vi "load_xml.vi"(8 "error in":errorcluster, 10 "child node in":refnum<k20>) -> (0 "error out":errorcluster, 2 "child node out":refnum<k20>, 3 "HSDIO Settings":T1={"Enable HSDIO Pulses"=TRUE, "Resource Name"="PXI1Slot6", "Clock Rate"=20000000.0, "Array of Script Triggers"=[], "Pulse Generation Script"="script script1\n     Generate RedTrap_compress_temp\nend script", "Start Trigger"={"Wait for start trigger?"=FALSE, "source (PFI 0)"="PFI0", "edge (rising)"=12}, "Hardware alignment quantum\n(in samples)"=1, "Inital State"="", "Idle State"="", "Active Channels"="", "Array of Waveforms"=[]} {"Hardware alignment quantum\n(in samples)" min=1 step=1; "Array of Script Triggers"."level" items=["High Level"=34, "Low Level"=35]; "Array of Script Triggers"."edge" items=["Rising Edge"=12, "Falling Edge"=13]; "Start Trigger"."edge (rising)" items=["Rising Edge"=12, "Falling Edge"=13]; "Clock Rate" min=0.0 max=200000000.0 format="%.2p"})   [LabVIEW 2013, in "HSDIO.lvclass"]
doc: "Loads HSDIO settings from xml. Expected format:\n\n<EnableHSDIOPulses>%b</EnableHSDIOPulses>\n<ResourceName>%s</ResourceName>\n<ClockRate>%f</ClockRate>\n<unitsPerSecond>%f</unitsPerSecond>\n<HardwareAlignmentQuantum units=\"samples\">%u</HardwareAlignmentQuantum>\n<ArrayOfScriptTriggers columns=\"id, source, type, edge, level\">\n<trigger>%s\\t%s\\t%s\\t%s\\t%s</trigger>\n</ArrayOfScriptTriggers>\n<ChannelsControl columns=\"Description, Active?, Idle State\">\n<channel>%s</channel>\n</ChannelsControl>\n<PulseGenerationScript>%s</PulseGenerationScript>\n<DirectoryToLookForWaveformFiles>%s</DirectoryToLookForWaveformFiles>\n<StartTrigger.WaitForStartTrigger>%b</StartTrigger.WaitForStartTrigger>\n<StartTrigger.source>%s</StartTrigger.source>\n<StartTrigger.edge>%s</StartTrigger.edge>\n\nMTL 2013 Jan 1"
uses:
  HSDIO.lvclass
  <resource>/objmgr/DOMUserDefRef.rc
  <vilib>/xml/NI_XML.lvlib
  <vilib>/xml/Close Reference(Node).vi
  <instrlib>/niHSDIO/niHSDIO.llb/niHSDIO_ctl Trigger Script - trigID Values (Ring).ctl
  <instrlib>/niHSDIO/niHSDIO.llb/niHSDIO_ctl Trigger Source Values (Ring).ctl
  <instrlib>/niHSDIO/niHSDIO.llb/niHSDIO_ctl Trigger DigEdge - Edge Values (Ring).ctl
  <instrlib>/niHSDIO/niHSDIO.llb/niHSDIO_ctl Trigger DigLvl - Level Values (Ring).ctl
  HSDIO_settings.ctl
  waveform.ctl
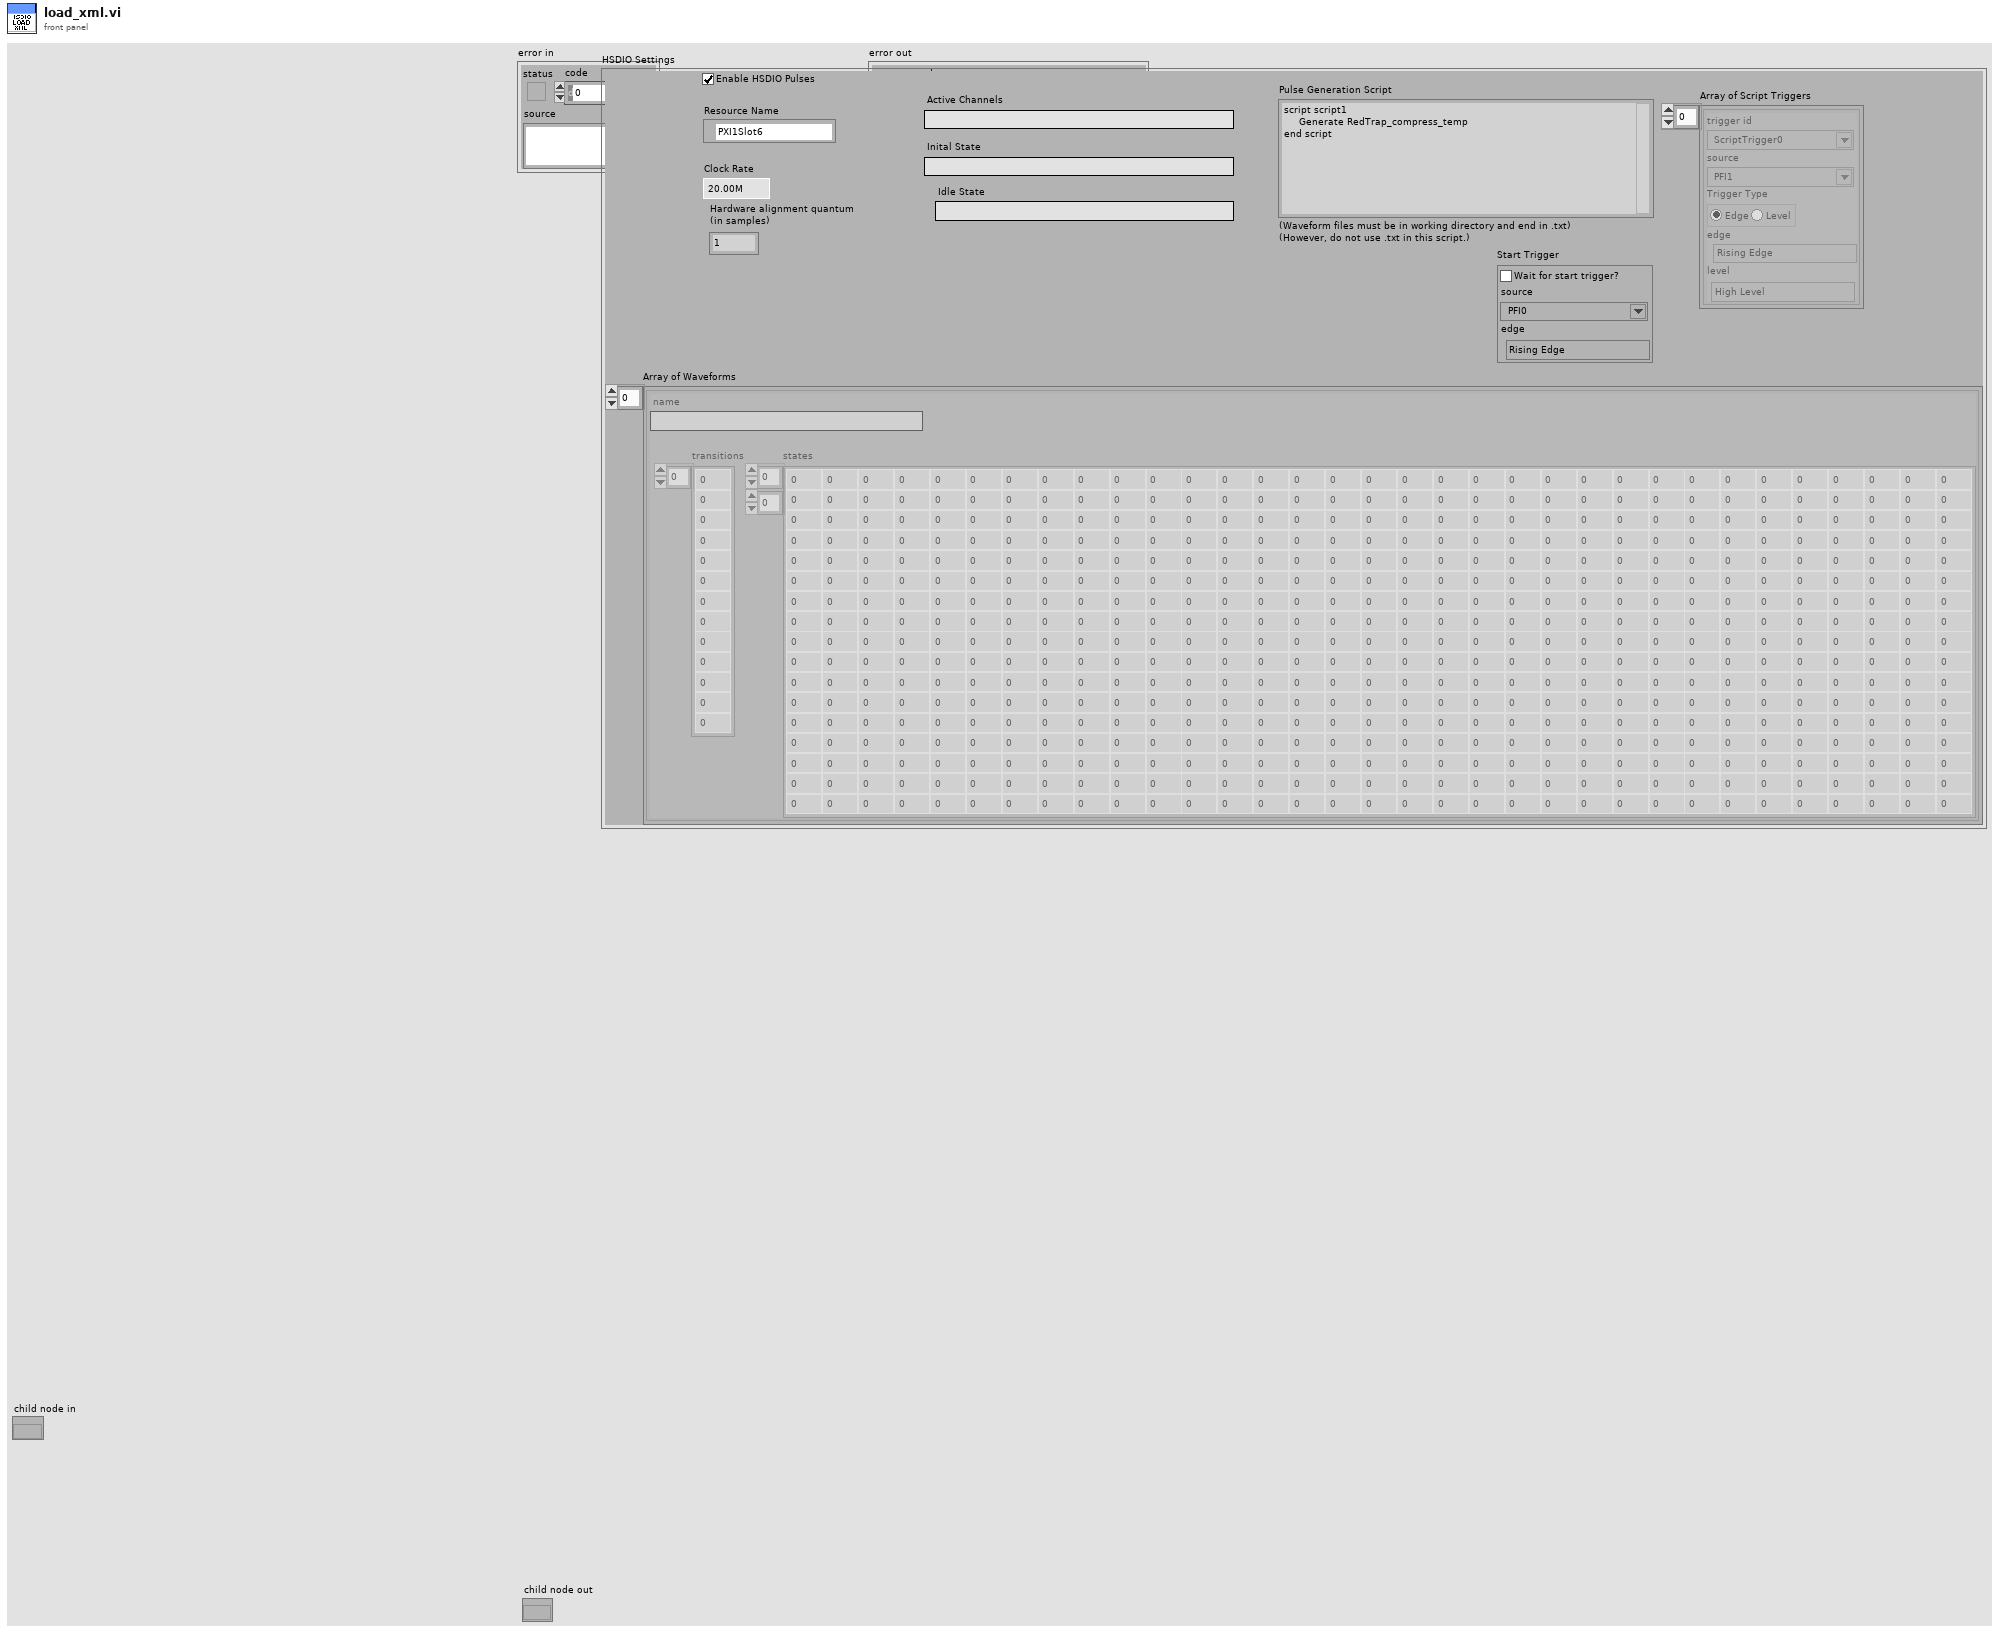
[diagram p1: front panel]
types:
  T1 = typedef "HSDIO.lvclass/HSDIO_settings.ctl" = cluster{"Enable HSDIO Pulses":bool, "Resource Name":refnum<k15>, "Clock Rate":dbl, "Array of Script Triggers":cluster{"trigger id (script trigger 0)":T2, "source (PFI 0)":T3, "Trigger Type":enum32{"Edge", "Level"}, "edge":T4, "level":T5}[], "Pulse Generation Script":string, "Start Trigger":cluster{"Wait for start trigger?":bool, "source (PFI 0)":T3, "edge (rising)":T4}, "Hardware alignment quantum\n(in samples)":u16, "Inital State":string, "Idle State":string, "Active Channels":string, "Array of Waveforms":T6[]}
  T2 = typedef "niHSDIO_ctl Trigger Script - trigID Values (Ring).ctl" = string
  T3 = typedef "niHSDIO_ctl Trigger Source Values (Ring).ctl" = string
  T4 = typedef "niHSDIO_ctl Trigger DigEdge - Edge Values (Ring).ctl" = i32
  T5 = typedef "niHSDIO_ctl Trigger DigLvl - Level Values (Ring).ctl" = i32
  T6 = typedef "HSDIO.lvclass/waveform.ctl" = cluster{"name":string, "transitions":u32[], "states":u8[][]}
  T7 = cluster{"trigger id (script trigger 0)":T2, "source (PFI 0)":T3, "Trigger Type":enum32{"Edge", "Level"}, "edge":T4, "level":T5}
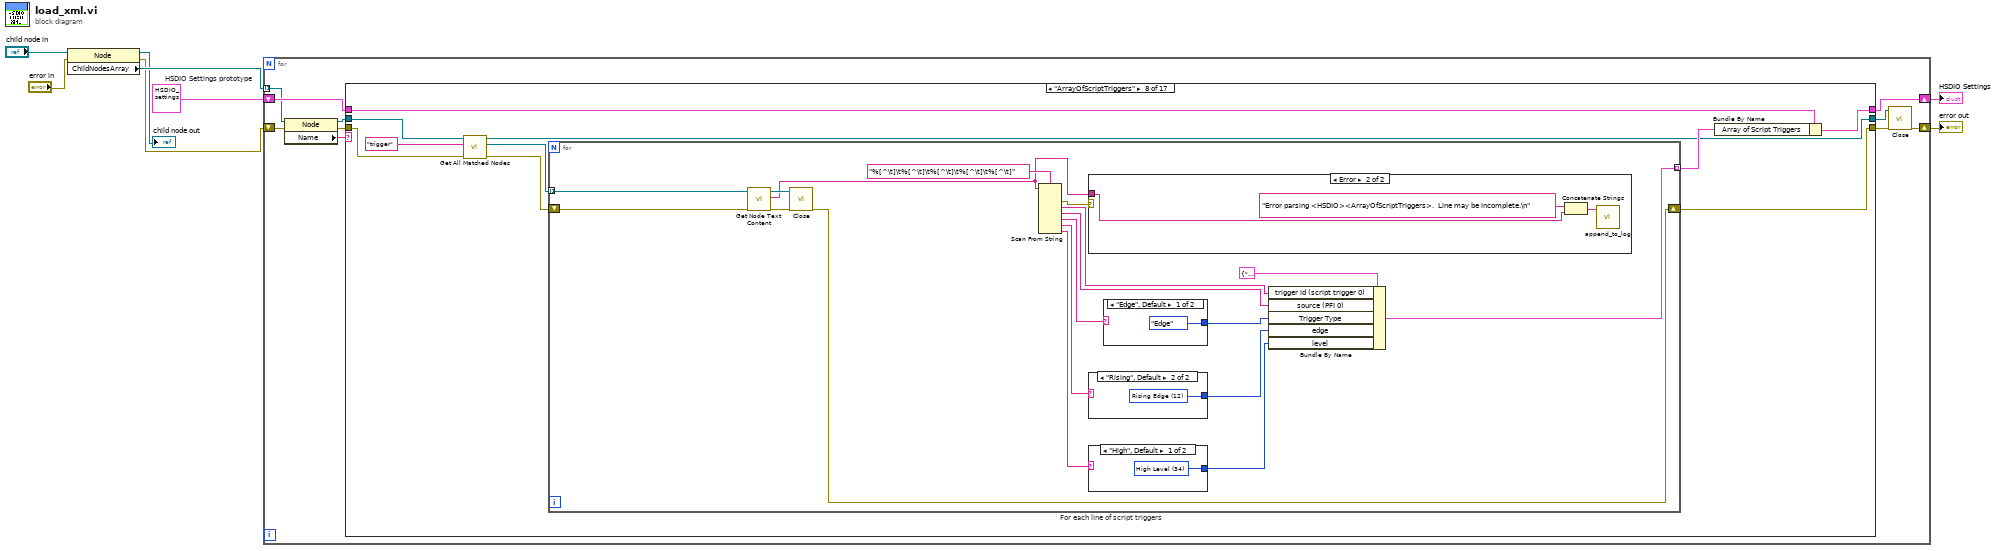
[diagram p0: block diagram]
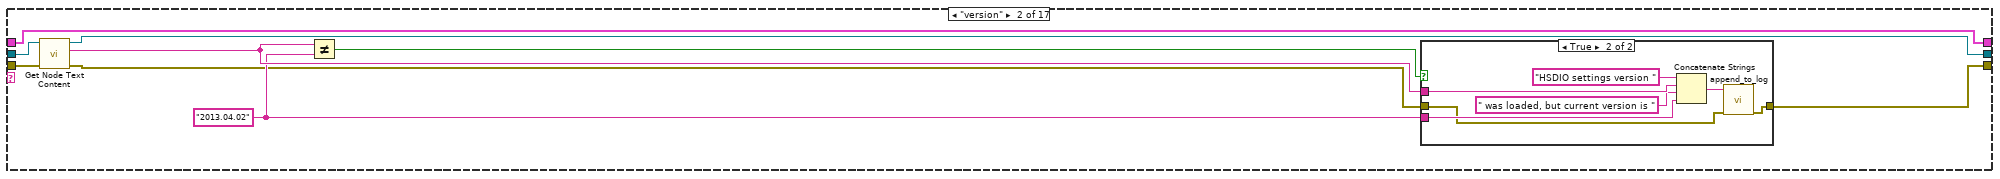
[diagram p3: hidden frame]
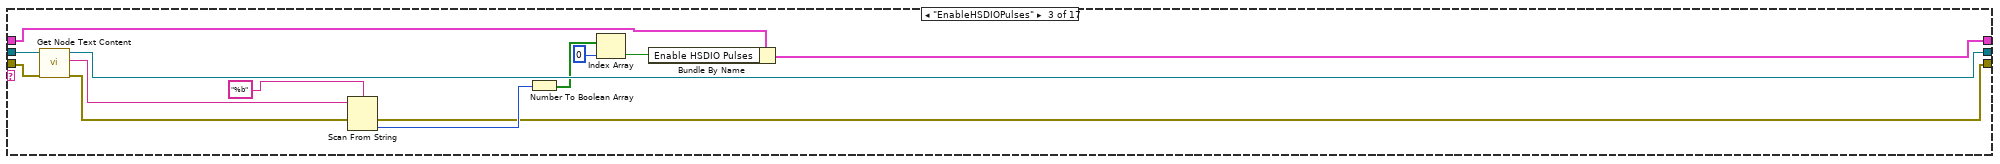
[diagram p5: hidden frame]
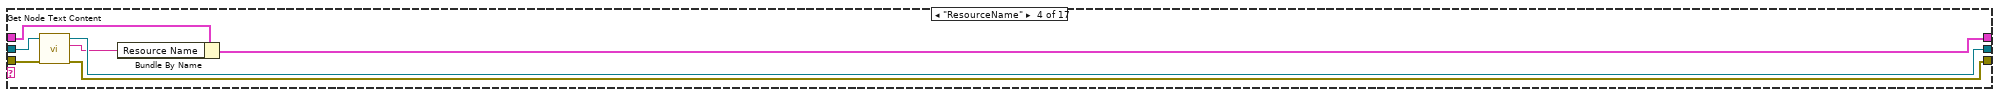
[diagram p6: hidden frame]
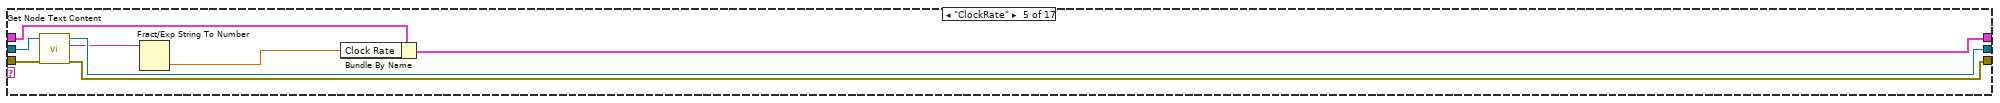
[diagram p7: hidden frame]
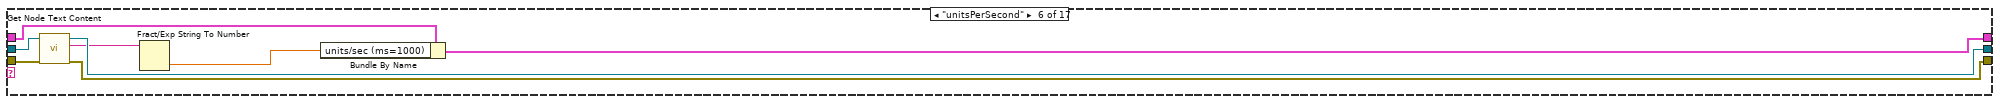
[diagram p8: hidden frame]
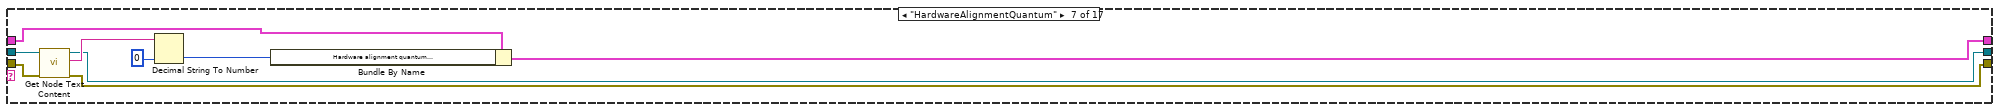
[diagram p9: hidden frame]
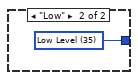
[diagram p10: hidden frame]
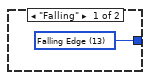
[diagram p11: hidden frame]
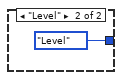
[diagram p12: hidden frame]
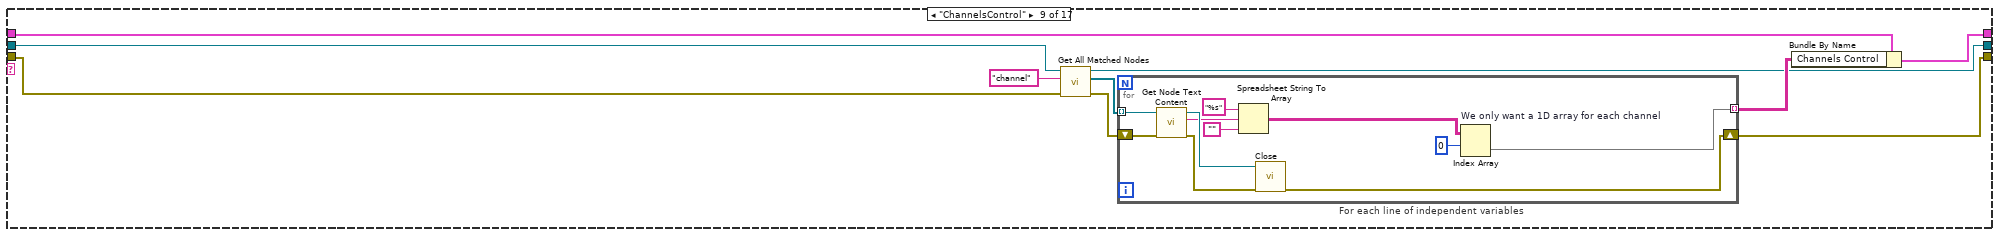
[diagram p14: hidden frame]
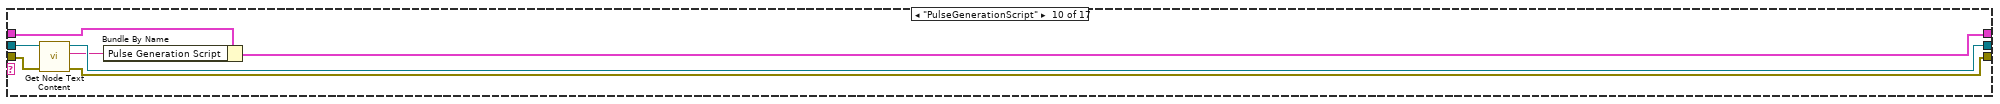
[diagram p15: hidden frame]
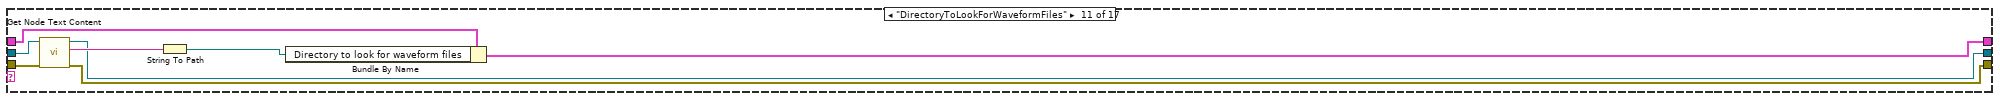
[diagram p16: hidden frame]
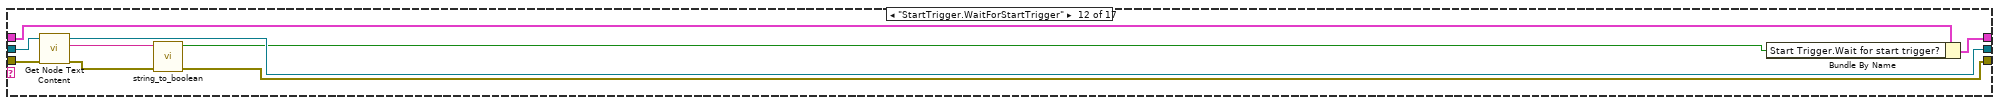
[diagram p17: hidden frame]
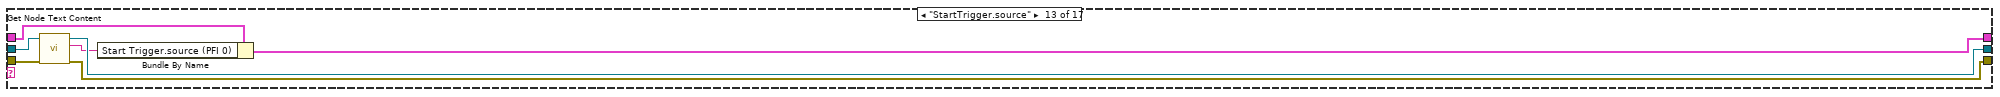
[diagram p18: hidden frame]
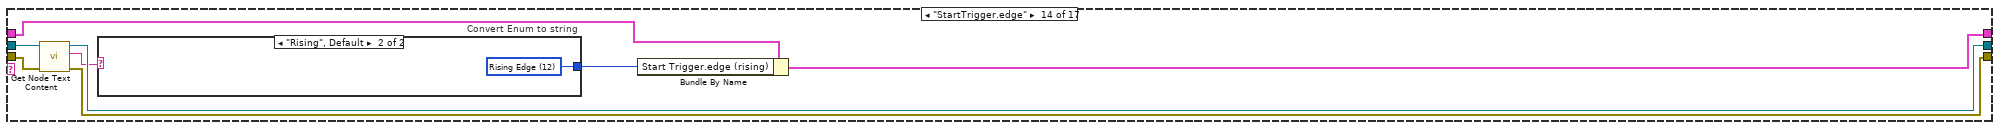
[diagram p19: hidden frame]
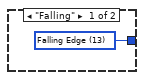
[diagram p20: hidden frame]
diagram:
  w3 = T1 {"Enable HSDIO Pulses"=FALSE, "Resource Name"="", "Clock Rate"=0.0, "Array of Script Triggers"=[], "Pulse Generation Script"="", "Start Trigger"={"Wait for start trigger?"=FALSE, "source (PFI 0)"="", "edge (rising)"=0}, "Hardware alignment quantum\n(in samples)"=0, "Inital State"="", "Idle State"="", "Active Channels"="", "Array of Waveforms"=[]}  # HSDIO Settings prototype
  n1 = property class="Node"(reference="child node in", error in="error in") -> (reference out=→"child node out":refnum<k20>, error out=w6:errorcluster, "ChildNodesArray"=w8:refnum<k20>[])
  n2 = for {
    tunnel: w8 -> [w10] mode=indexing
    shift-right: [w15] -> w4
    shift-left: w3 -> [w16]
    shift-right: [w12] -> w2
    shift-left: w6 -> [w9]
    n3 = property class="Node"(reference=w10, error in=w9) -> (reference out=w17:refnum<k20>, error out=w13:errorcluster, "Name"=w18:string)
    n4 = case shown="\"ArrayOfScriptTriggers\"" w18 {
      tunnel: w17 -> [w20 w26 w50 w55 w63 w71 w79 w93 w130 w145 w151 w164 w169 w177 w190 w194 w203]
      tunnel: w16 -> [w21 w24 w40 w58 w66 w74 w83 w90 w127 w148 w156 w162 w172 w180 w188 w199 w206]
      tunnel: [w21 w24 w39 w57 w65 w73 w82 w88 w125 w147 w155 w161 w171 w179 w187 w198 w205] -> w15
      tunnel: [w20 w23 w51 w56 w64 w72 w78 w87 w124 w146 w152 w165 w170 w178 w191 w195 w204] -> w14
      tunnel: w13 -> [w19 w25 w49 w54 w62 w70 w77 w86 w123 w144 w150 w163 w168 w176 w189 w193 w202]
      tunnel: [w19 w22 w41 w53 w61 w69 w76 w84 w121 w143 w149 w157 w167 w175 w183 w192 w201] -> w11
      frame "None", Default {
      }
      frame "version" {
        w28 = "2013.04.02" ("y")
        n5 = call <vilib>:"Get Node Text Content.vi"("error in (no error)"=w25, "node in"=w26) -> ("error out"=w27:errorcluster, "node text"=w29:string, "node out"=w23:refnum<k20>)  [unwired: 7 in]
        n6 = Not Equal?(x=w29, y=w28) -> (x != y?=w30:bool)
        n7 = case shown="True" w30 {
          tunnel: w29 -> [_ w37]
          tunnel: w28 -> [_ w35]
          tunnel: w27 -> [w31 w33]
          tunnel: [w31 w32] -> w22
          frame False {
          }
          frame True {
            n8 = Concatenate Strings("HSDIO settings version " ("string"), w37, " was loaded, but current version is " ("string"), w35) -> (w34:string)
            n9 = call "append_to_log.vi"("error in"=w33, "string"=w34) -> ("error out"=w32:errorcluster)  [unwired: 9 in]
          }
        }
      }
      frame "EnableHSDIOPulses" {
        n10 = call <vilib>:"Get Node Text Content.vi"("error in (no error)"=w49, "node in"=w50) -> ("error out"=w42:errorcluster, "node text"=w43:string, "node out"=w51:refnum<k20>)  [unwired: 7 in]
        n11 = Scan From String(format string="%b", input string=w43, error in=w42) -> (error out=w41:errorcluster, output 1=w44:i32)  [unwired: 2 in, 2 out]
        n12 = Number To Boolean Array(number=w44) -> (Boolean array=w48:bool[])
        n13 = Index Array(array=w48, index=0) -> (element=w46:bool)
        n14 = Bundle By Name(cluster=w40, "Enable HSDIO Pulses"=w46) -> (w39:T1)
      }
      frame "ResourceName" {
        n15 = call <vilib>:"Get Node Text Content.vi"("error in (no error)"=w54, "node in"=w55) -> ("error out"=w53:errorcluster, "node text"=w52:string, "node out"=w56:refnum<k20>)  [unwired: 7 in]
        n16 = Bundle By Name(cluster=w58, "Resource Name"=w52) -> (w57:T1)
      }
      frame "ClockRate" {
        n17 = call <vilib>:"Get Node Text Content.vi"("error in (no error)"=w62, "node in"=w63) -> ("error out"=w61:errorcluster, "node text"=w60:string, "node out"=w64:refnum<k20>)  [unwired: 7 in]
        n18 = Fract/Exp String To Number(string=w60) -> (number=w59:dbl)  [unwired: 3 in, 1 out]
        n19 = Bundle By Name(cluster=w66, "Clock Rate"=w59) -> (w65:T1)
      }
      frame "unitsPerSecond" {
        n20 = call <vilib>:"Get Node Text Content.vi"("error in (no error)"=w70, "node in"=w71) -> ("error out"=w69:errorcluster, "node text"=w68:string, "node out"=w72:refnum<k20>)  [unwired: 7 in]
        n21 = Fract/Exp String To Number(string=w68) -> (number=w67:dbl)  [unwired: 3 in, 1 out]
        n22 = Bundle By Name(cluster=w74, "units/sec (ms=1000)"=w67) -> (w73:T1)
      }
      frame "HardwareAlignmentQuantum" {
        n23 = call <vilib>:"Get Node Text Content.vi"("error in (no error)"=w77, "node in"=w79) -> ("error out"=w76:errorcluster, "node text"=w81:string, "node out"=w78:refnum<k20>)  [unwired: 7 in]
        n24 = Decimal String To Number(string=w81, default (0L)=u16 0 ("default (0 I32)")) -> (number=w80:u16)  [unwired: 1 in, 1 out]
        n25 = Bundle By Name(cluster=w83, "Hardware alignment quantum\n(in samples)"=w80) -> (w82:T1)
      }
      frame "ArrayOfScriptTriggers" {
        n26 = call <vilib>:"Get All Matched Nodes.vi"("error in (no error)"=w86, "XPath expression"="trigger", "node in"=w93) -> ("error out"=w85:errorcluster, "node result array"=w91:refnum<k20>[], "node out"=w87:refnum<k20>)  [unwired: 6 in]
        n27 = for "For each line of script triggers" {
          tunnel: w91 -> [w109] mode=indexing
          tunnel: [w110] -> w89 mode=indexing
          shift-right: [w106] -> w84
          shift-left: w85 -> [w107]
          n28 = call <vilib>:"Get Node Text Content.vi"("error in (no error)"=w107, "node in"=w109) -> ("error out"=w98:errorcluster, "node text"=w94:string, "node out"=w108:refnum<k20>)  [unwired: 7 in]
          n29 = call-poly <vilib>:"Close.vi"("error in (no error)"=w98, "node"=w108) -> ("error out"=w106:errorcluster)  [unwired: 7 in]
          n30 = Scan From String(format string="%[^\t]\t%[^\t]\t%[^\t]\t%[^\t]\t%[^\t]", input string=w94) -> (error out=w95:errorcluster, output 1=w97:string, output 2=w96:string, output 3=w105:string, output 4=w103:string, output 5=w101:string)  [unwired: 7 in, 2 out]
          n31 = case shown="Error" w95 {
            tunnel: w94 -> [_ w118]
            frame No Error {
            }
            frame Error {
              n32 = Concatenate Strings("Error parsing <HSDIO><ArrayOfScriptTriggers>.  Line may be incomplete.\n" ("string"), w118) -> (w119:string)
              n33 = call "append_to_log.vi"("string"=w119) -> ()  [unwired: 10 in, 1 out]
            }
          }
          n34 = case shown="\"Rising\", Default" w103 {
            tunnel: [w114 w115] -> w102
            frame "Falling" {
              w114 = T4 13 items=["Rising Edge"=12, "Falling Edge"=13] ("edge")
            }
            frame "Rising", Default {
              w115 = T4 12 items=["Rising Edge"=12, "Falling Edge"=13] ("edge")
            }
          }
          n35 = case shown="\"High\", Default" w101 {
            tunnel: [w112 w113] -> w100
            frame "High", Default {
              w112 = T5 34 items=["High Level"=34, "Low Level"=35] ("level")
            }
            frame "Low" {
              w113 = T5 35 items=["High Level"=34, "Low Level"=35] ("level")
            }
          }
          n36 = case shown="\"Edge\", Default" w105 {
            tunnel: [enum32{"Edge", "Level"}."Edge" ("Trigger Type") enum32{"Edge", "Level"}."Level" ("Trigger Type")] -> w104
            frame "Edge", Default {
            }
            frame "Level" {
            }
          }
          n37 = Bundle By Name(cluster=T7 {"trigger id (script trigger 0)"="", "source (PFI 0)"="", "Trigger Type"=enum."Edge", "edge"=0, "level"=0} ("Script Trigger"), "trigger id (script trigger 0)"=w97, "source (PFI 0)"=w96, "Trigger Type"=w104, "edge"=w102, "level"=w100) -> (w110:T7)
        }
        n38 = Bundle By Name(cluster=w90, "Array of Script Triggers"=w89) -> (w88:T1)
      }
      frame "ChannelsControl" {
        n39 = call <vilib>:"Get All Matched Nodes.vi"("error in (no error)"=w123, "XPath expression"="channel", "node in"=w130) -> ("error out"=w122:errorcluster, "node result array"=w128:refnum<k20>[], "node out"=w124:refnum<k20>)  [unwired: 6 in]
        n40 = for "For each line of independent variables" {
          tunnel: w128 -> [w141] mode=indexing
          tunnel: [w131] -> w126 mode=indexing
          shift-right: [w138] -> w121
          shift-left: w122 -> [w139]
          n41 = call <vilib>:"Get Node Text Content.vi"("error in (no error)"=w139, "node in"=w141) -> ("error out"=w137:errorcluster, "node text"=w132:string, "node out"=w140:refnum<k20>)  [unwired: 7 in]
          n42 = Spreadsheet String To Array(format string="%s", spreadsheet string=w132, array type (2D Dbl)="") -> (array=w134:string[][])  [unwired: 1 in]
          n43 = call-poly <vilib>:"Close.vi"("error in (no error)"=w137, "node"=w140) -> ("error out"=w138:errorcluster)  [unwired: 7 in]
          n44 = Index Array "We only want a 1D array for each channel"(array=w134, index (row)=0) -> (element=w131:string[])  [unwired: 1 in]
        }
        n45 = Bundle By Name(cluster=w127, "Channels Control"=w126) -> (w125:T1)
      }
      frame "PulseGenerationScript" {
        n46 = call <vilib>:"Get Node Text Content.vi"("error in (no error)"=w144, "node in"=w145) -> ("error out"=w143:errorcluster, "node text"=w142:string, "node out"=w146:refnum<k20>)  [unwired: 7 in]
        n47 = Bundle By Name(cluster=w148, "Pulse Generation Script"=w142) -> (w147:T1)
      }
      frame "DirectoryToLookForWaveformFiles" {
        n48 = call <vilib>:"Get Node Text Content.vi"("error in (no error)"=w150, "node in"=w151) -> ("error out"=w149:errorcluster, "node text"=w154:string, "node out"=w152:refnum<k20>)  [unwired: 7 in]
        n49 = String To Path(string=w154) -> (path=w153:path)
        n50 = Bundle By Name(cluster=w156, "Directory to look for waveform files"=w153) -> (w155:T1)
      }
      frame "StartTrigger.WaitForStartTrigger" {
        n51 = call <vilib>:"Get Node Text Content.vi"("error in (no error)"=w163, "node in"=w164) -> ("error out"=w158:errorcluster, "node text"=w160:string, "node out"=w165:refnum<k20>)  [unwired: 7 in]
        n52 = call "string_to_boolean.vi"("error in"=w158, "string"=w160) -> ("error out"=w157:errorcluster, "boolean"=w159:bool)  [unwired: 8 in]
        n53 = Bundle By Name(cluster=w162, "Start Trigger.Wait for start trigger?"=w159) -> (w161:T1)
      }
      frame "StartTrigger.source" {
        n54 = call <vilib>:"Get Node Text Content.vi"("error in (no error)"=w168, "node in"=w169) -> ("error out"=w167:errorcluster, "node text"=w166:string, "node out"=w170:refnum<k20>)  [unwired: 7 in]
        n55 = Bundle By Name(cluster=w172, "Start Trigger.source (PFI 0)"=w166) -> (w171:T1)
      }
      frame "StartTrigger.edge" {
        n56 = call <vilib>:"Get Node Text Content.vi"("error in (no error)"=w176, "node in"=w177) -> ("error out"=w175:errorcluster, "node text"=w174:string, "node out"=w178:refnum<k20>)  [unwired: 7 in]
        n57 = case "Convert Enum to string" shown="\"Rising\", Default" w174 {
          tunnel: [w181 w182] -> w173
          frame "Falling" {
            w181 = T4 13 items=["Rising Edge"=12, "Falling Edge"=13] ("Start Trigger.edge (rising)")
          }
          frame "Rising", Default {
            w182 = T4 12 items=["Rising Edge"=12, "Falling Edge"=13] ("Start Trigger.edge (rising)")
          }
        }
        n58 = Bundle By Name(cluster=w180, "Start Trigger.edge (rising)"=w173) -> (w179:T1)
      }
      frame "UseFileScript" {
        n59 = call <vilib>:"Get Node Text Content.vi"("error in (no error)"=w189, "node in"=w190) -> ("error out"=w184:errorcluster, "node text"=w186:string, "node out"=w191:refnum<k20>)  [unwired: 7 in]
        n60 = call "string_to_boolean.vi"("error in"=w184, "string"=w186) -> ("error out"=w183:errorcluster, "boolean"=w185:bool)  [unwired: 8 in]
        n61 = Bundle By Name(cluster=w188, "Use file script"=w185) -> (w187:T1)
      }
      frame "BasePathForScript" {
        n62 = call <vilib>:"Get Node Text Content.vi"("error in (no error)"=w193, "node in"=w194) -> ("error out"=w192:errorcluster, "node text"=w197:string, "node out"=w195:refnum<k20>)  [unwired: 7 in]
        n63 = String To Path(string=w197) -> (path=w196:path)
        n64 = Bundle By Name(cluster=w199, "Base path for script"=w196) -> (w198:T1)
      }
      frame "FileNameForScript" {
        n65 = call <vilib>:"Get Node Text Content.vi"("error in (no error)"=w202, "node in"=w203) -> ("error out"=w201:errorcluster, "node text"=w200:string, "node out"=w204:refnum<k20>)  [unwired: 7 in]
        n66 = Bundle By Name(cluster=w206, "filename for script"=w200) -> (w205:T1)
      }
    }
    n67 = call-poly <vilib>:"Close.vi"("error in (no error)"=w11, "node"=w14) -> ("error out"=w12:errorcluster)  [unwired: 7 in]
  }
  "error out" <- w2
  "HSDIO Settings" <- w4
